vi "svfa_Window Frequency Response (first derivative).vi"   [LabVIEW 2017]
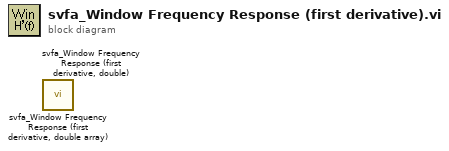
[diagram p0: block diagram]
diagram:
  n1 = call <vilib>:"svfa_Window Frequency Response (first derivative, double array).vi"() -> ()  [unwired: 3 in, 1 out]
  n2 = call <vilib>:"svfa_Window Frequency Response (first derivative, double).vi"() -> ()  [unwired: 3 in, 1 out]
